vi "Match.vi"(10 "log record":T1 {"timestamp" format="%<%x %.3X>T"}, 11 "filter in":refnum<class "Filter.lvclass">) -> (2 "matches":bool[](array[boolean]), 3 "filter out":refnum<class "Filter.lvclass">)   [LabVIEW 2018, in "GLog.lvlib" / "Filter.lvclass"]
uses:
  Filter.lvclass
  logger_class/Log Record.ctl
  logger_class/Internal Log Levels.ctl
  logger_class/Logger.lvclass
panel:
  # "Connector Pane"
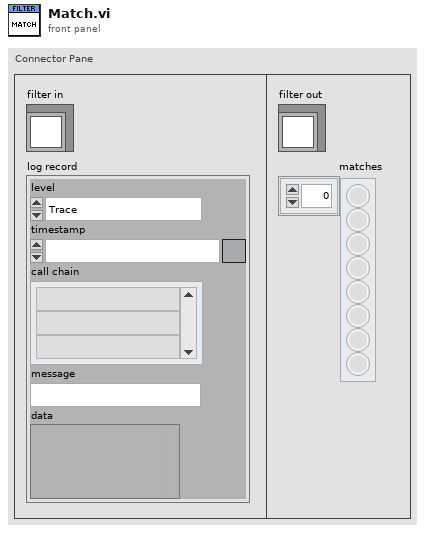
[diagram p1: front panel]
types:
  T1 = typedef "GLog.lvlib/Logger.lvclass/Log Record.ctl" = cluster{"level":T2, "timestamp":timestamp, "call chain":string[], "message":string, "data":variant}
  T2 = typedef "GLog.lvlib/Logger.lvclass/Internal Log Levels.ctl" = enum16{"Trace", "Debug", "Info", "Warning", "Error", "Critical", "Internal"}
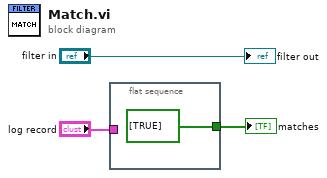
[diagram p0: block diagram]
diagram:
  n1 = flat-sequence {
    tunnel: [bool[] [TRUE]] -> w2
    tunnel: "log record" -> [_]
    frame #0 {
    }
  }
  "filter out" <- "filter in"
  "matches" <- w2
